vi "get_grouppath_exp.vi"(0 "Experiment.lvclass in":refnum<class "Experiment.lvclass">, 1 "error in (no error)":errorcluster) -> (2 "GroupPath":path, 3 "Experiment.lvclass out":refnum<class "Experiment.lvclass">, 4 "error out":errorcluster)   [LabVIEW 2015, in "Experiment.lvclass"]
uses:
  Experiment.lvclass
  Experiment.lvclass/Experiment.ctl
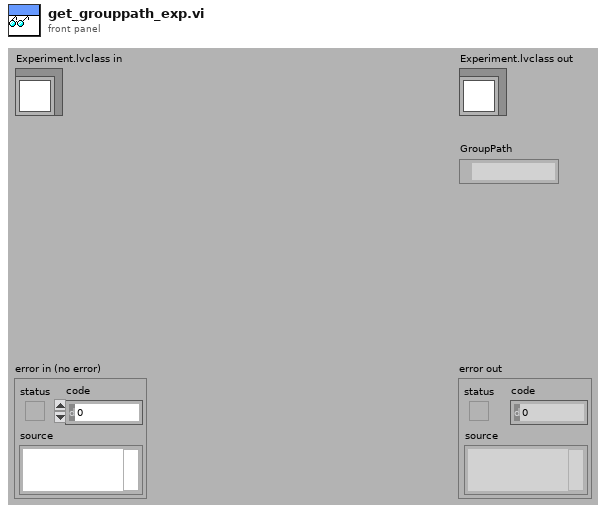
[diagram p1: front panel]
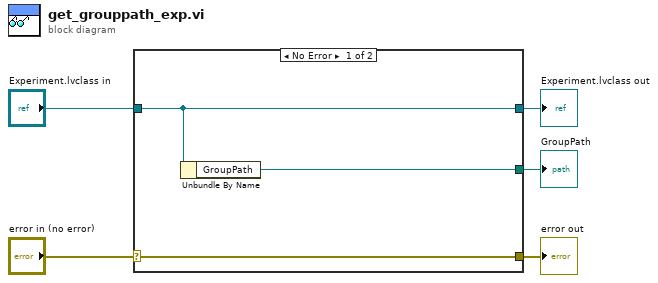
[diagram p0: block diagram]
diagram:
  n1 = case shown="No Error" "error in (no error)" {
    selector: "error in (no error)" -> [w8 w9]
    tunnel: [w8 w9] -> w4
    tunnel: [w7 w10] -> w2
    tunnel: "Experiment.lvclass in" -> [w7 w10]
    tunnel: [w6 _] -> w1
    frame No Error {
      n2 = Unbundle By Name(w7) -> ("GroupPath"=w6:path)
    }
    frame Error {
    }
  }
  "error out" <- w4
  "Experiment.lvclass out" <- w2
  "GroupPath" <- w1
